vi "TDMSextractspreadsheet.vi"(11 "file path":path) -> (0 "channel list":string, 2 "dt":dbl, 3 "data":dbl[][](array[numeric]))   [LabVIEW 2015]
panel:
  in  "data type":waveform(dbl)[](array[waveform])
  out "channel aray":string[](array[string])
  out "group":string
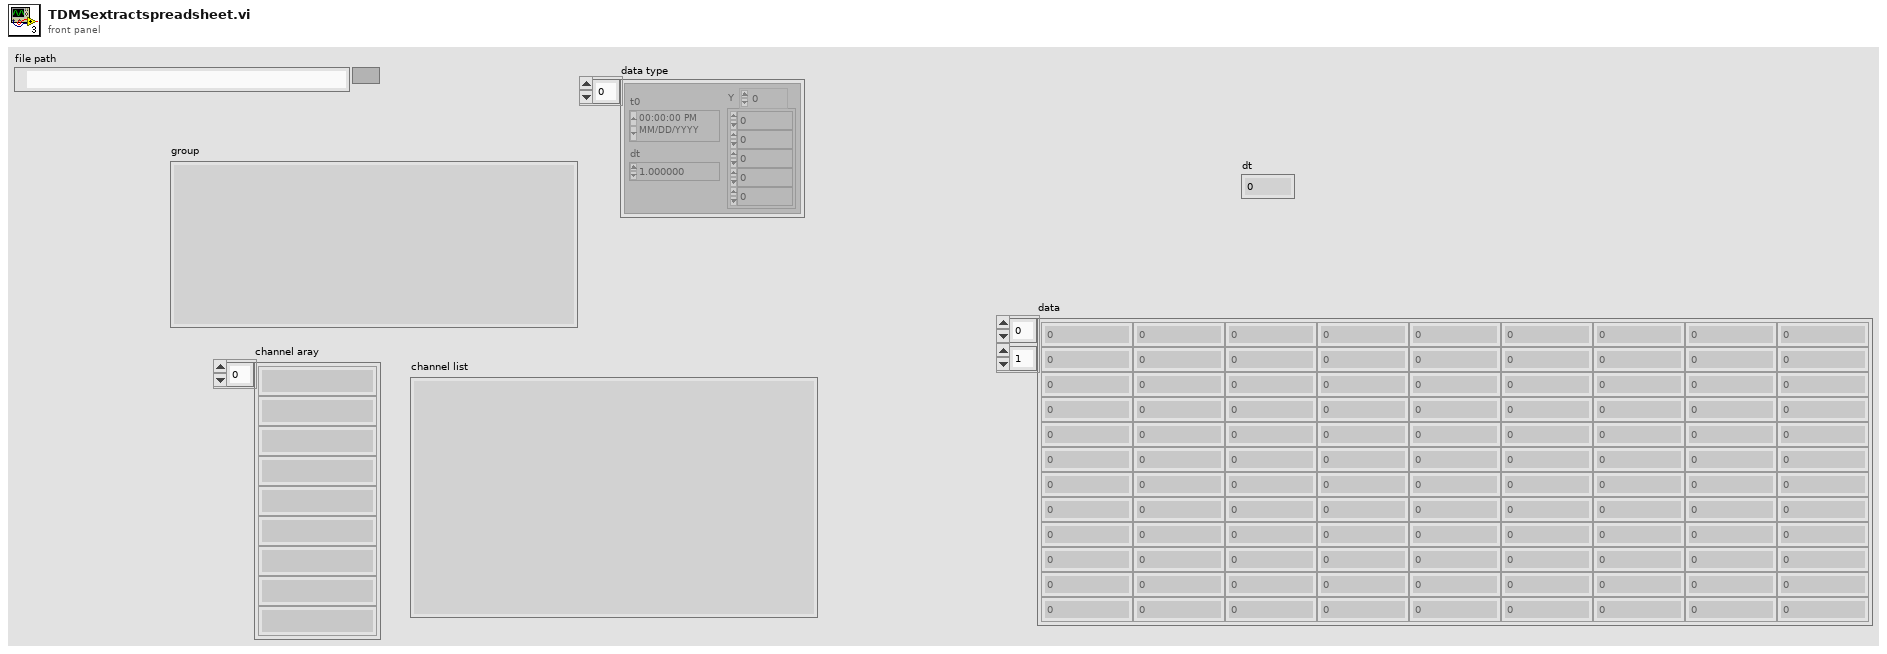
[diagram p1: front panel]
types:
  T1 = enum16{"open", "open or create", "create or replace", "create", "open (read-only)"}
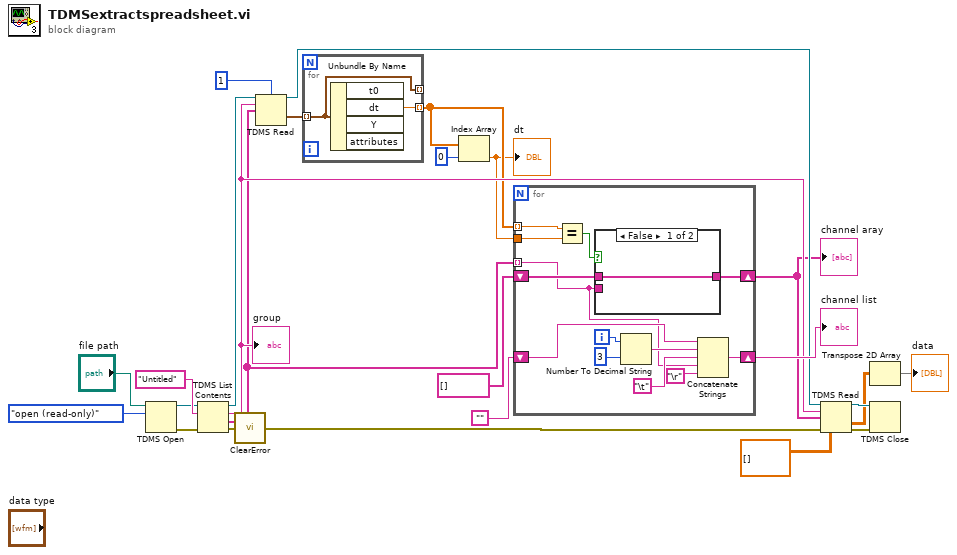
[diagram p0: block diagram]
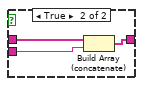
[diagram p2: hidden frame]
diagram:
  n1 = TDMS Open(10:T1."open (read-only)" ("operation (0:open)"), 11:"file path") -> (0:w17:errorcluster, 3:w24:refnum<k34>)  [unwired: 5 in]
  n2 = TDMS List Contents(4:w17, 6:"Untitled" ("Group name"), 7:w24) -> (0:w1:errorcluster, 1:w7:string[], 2:w14:string, 3:w13:refnum<k34>)
  "group" <- w14
  n3 = call <vilib>:"ClearError.vi"("error in (no error)"=w1) -> ("error out"=w16:errorcluster)
  n4 = TDMS Read(0:w13, 2:i64 1 ("count (-1: all)"), 5:w14, 7:w7) -> (4:w12:refnum<k34>, 10:w11:waveform(dbl)[])  [unwired: 4 in, 4 out]
  n5 = for {
    tunnel: [w26] -> _ mode=indexing
    tunnel: [w27] -> w9 mode=indexing
    tunnel: w11 -> [w26] mode=indexing
    n6 = Unbundle By Name(w26) -> ("dt"=w27:dbl)  [unwired: 3 out]
  }
  n7 = Index Array(array=w9, index=0) -> (element=w2:dbl)
  "dt" <- w2
  n8 = for {
    tunnel: w7 -> [w29] mode=indexing
    shift-right: [w39] -> w21
    shift-left: "" -> [w40]
    tunnel: w2 -> [w33]
    tunnel: w9 -> [w32] mode=indexing
    shift-right: [w28] -> w6
    shift-left: string[] [] -> [w30]
    i -> [w37]
    n9 = Equal?(x=w32, y=w33) -> (x = y?=w31:bool)
    n10 = case shown="False" w31 {
      tunnel: w30 -> [w41 w44]
      tunnel: w29 -> [_ w43]
      tunnel: [w41 w42] -> w28
      frame False {
      }
      frame True {
        n11 = Build Array (concatenate)(w44, w43) -> (w42:string[])
      }
    }
    n12 = Number To Decimal String(number=w37, width (-)=3) -> (decimal integer string=w35:string)
    n13 = Concatenate Strings(w40, w35, "\t", w29, "\r") -> (w39:string)
  }
  "channel aray" <- w6
  "channel list" <- w21
  n14 = TDMS Read(0:w12, 5:w14, 7:w6, 11:w16, 12:dbl[][] [] ("transposed array")) -> (4:w20:refnum<k34>, 10:w3:dbl[][], 15:w15:errorcluster)  [unwired: 3 in, 3 out]
  n15 = Transpose 2D Array(2D array=w3) -> (transposed array=→"data":dbl[][])
  n16 = TDMS Close(8:w15, 11:w20) -> ()  [unwired: 2 out]
